vi "Load Stage Positions.vi"() -> (0 "appended array":bool[](array[boolean]))   [LabVIEW 2014]
panel:
  in  "Boolean 3":bool
  in  "OK Button":bool
  in  "Boolean 4":bool
  in  "Boolean 2":bool
  in  "Boolean":bool
  # "Which stage positions would you like to load?"
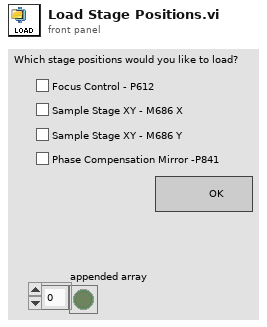
[diagram p1: front panel]
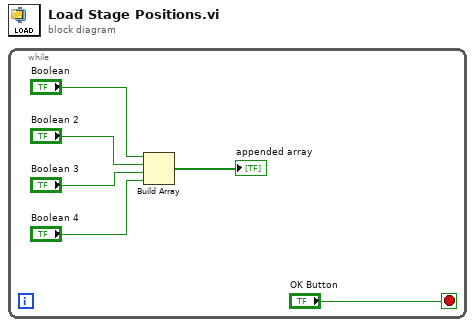
[diagram p0: block diagram]
diagram:
  n1 = while {
    stop <- "OK Button" stop-if-true
    n2 = Build Array("Boolean", "Boolean 2", "Boolean 3", "Boolean 4") -> (→"appended array":bool[])
  }
